vi "Get Error Handler.vi"(8 "error in (no error)":errorcluster, 11 "Asynchronous Action In":refnum<class "Async Action.lvclass">) -> (0 "error out":errorcluster, 2 "Error Handler":refnum<class "Error Handler Interface.lvclass">, 3 "Asynchronous Action Out":refnum<class "Async Action.lvclass">)   [LabVIEW 2020, in "Async Action.lvclass"]
doc: "Returns the error handler configured for the process using the Set Error Handler.vi method."
uses:
  Async Action.lvclass
  Error Handler Interface/Error Handler Interface.lvclass
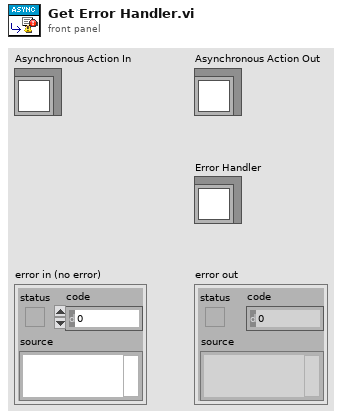
[diagram p1: front panel]
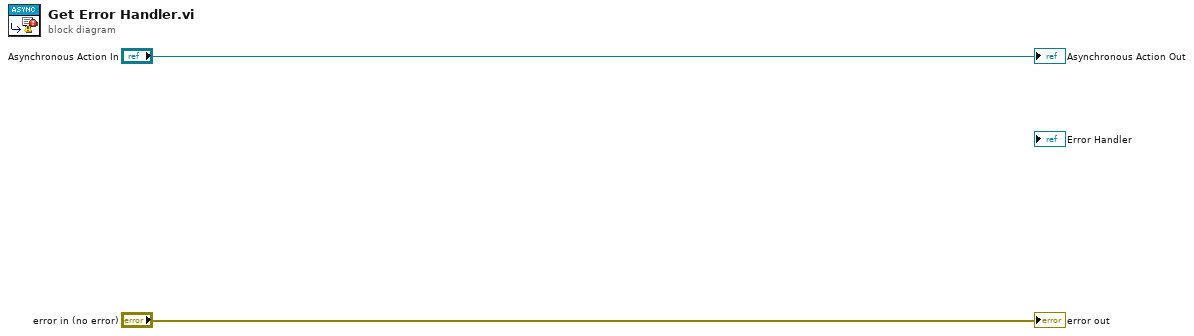
[diagram p0: block diagram]
diagram:
  "error out" <- "error in (no error)"
  "Asynchronous Action Out" <- "Asynchronous Action In"
